vi "Update Boolean from Ref.vi"(8 "error in (no error)":errorcluster, 10 "Boolean":bool, 11 "Boolean Ref in":refnum<vi>) -> (0 "error out":errorcluster, 3 "Boolean Ref out":refnum<vi>)   [LabVIEW 2024]
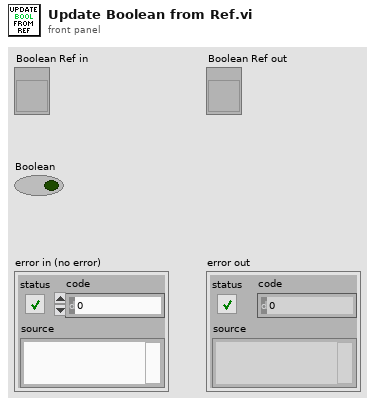
[diagram p1: front panel]
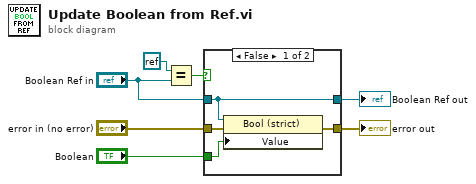
[diagram p0: block diagram]
diagram:
  n1 = Equal?(x=refnum<k0> refnum ("Not a Refnum Constant"), y="Boolean Ref in") -> (x = y?=w5:bool)
  n2 = case shown="False" w5 {
    tunnel: "Boolean Ref in" -> [w9 w12]
    tunnel: "Boolean" -> [w10 _]
    tunnel: [w9 w12] -> w2
    tunnel: [w11 w13] -> w7
    tunnel: "error in (no error)" -> [w8 w13]
    frame False {
      n3 = property on="Property Node" class="Bool (strict)"(reference=w9, error in=w8, "Value"=w10) -> (error out=w11:errorcluster)  [unwired: 1 out]
    }
    frame True {
    }
  }
  "error out" <- w7
  "Boolean Ref out" <- w2
